vi "[RT]Loop_Display.vi"   [LabVIEW 2018]
uses:
  [GlobVar]SensorState.vi
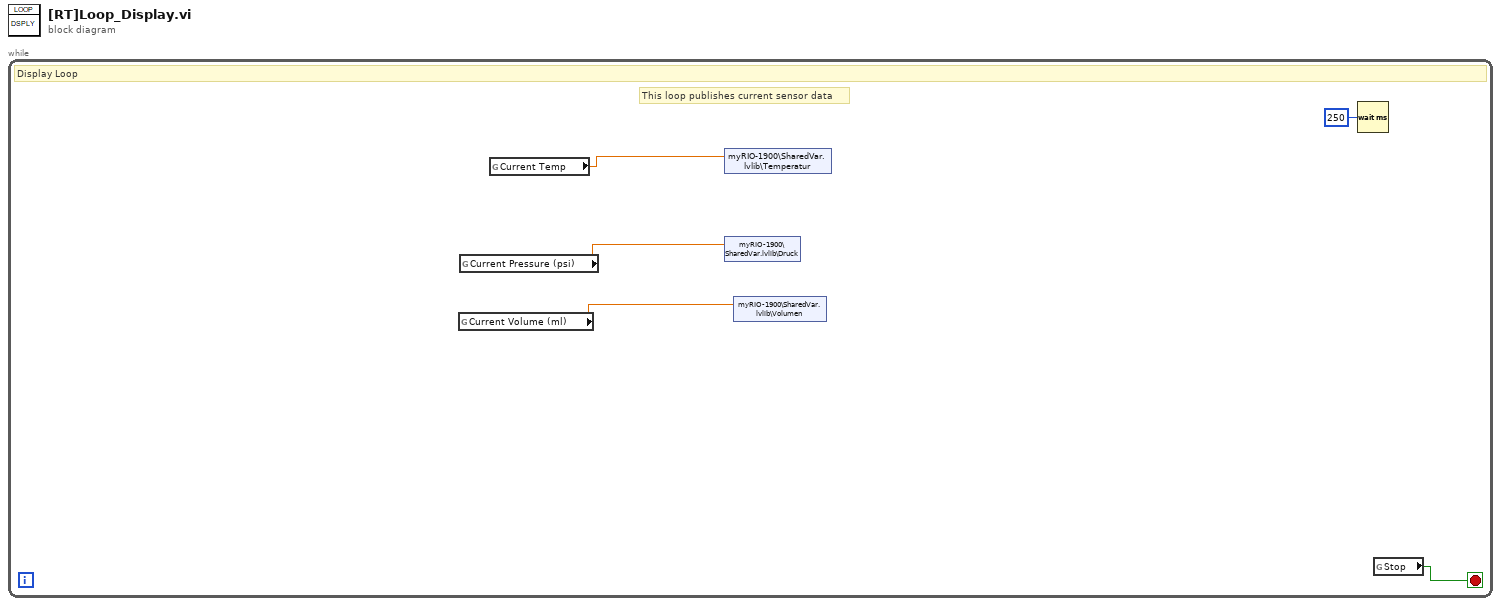
[diagram p0: block diagram]
diagram:
  n1 = while {
    stop <- w2 stop-if-true
    # "This loop publishes current sensor data"
    # "Display Loop"
    n2 = global read "[GlobVar]SensorState.vi" "Current Volume (ml)"() -> (w1:dbl)
    n3 = global read "[GlobVar]SensorState.vi" "Current Pressure (psi)"() -> (w3:dbl)
    n4 = global read "[GlobVar]SensorState.vi" "Current Temp"() -> (w5:dbl)
    n5 = shared-variable "myRIO-1900\\SharedVar.lvlib\\Temperatur"(w5) -> ()  [unwired: 1 in, 1 out]
    n6 = shared-variable "myRIO-1900\\SharedVar.lvlib\\Druck"(w3) -> ()  [unwired: 1 in, 1 out]
    n7 = shared-variable "myRIO-1900\\SharedVar.lvlib\\Volumen"(w1) -> ()  [unwired: 1 in, 1 out]
    n8 = Wait (ms)(milliseconds to wait=u32 250) -> ()  [unwired: 1 out]
    n9 = global read "[GlobVar]SensorState.vi" "Stop"() -> (w2:bool)
  }
